vi "Commit Hardware Relay State.vi"(0 "RelayInterface in":refnum<class "RelayInterface.lvclass">, 5 "Session Handle in":T1, 11 "error in (no error)":errorcluster) -> (4 "RelayInterface out":refnum<class "RelayInterface.lvclass">, 15 "error out":errorcluster)   [LabVIEW 2015, in "RelayInterface.lvclass"]
uses:
  RelayInterface.lvclass
  SLSC Session/Typedefs/Session Handle.ctl
  SLSC Session/SLSC Session.lvclass
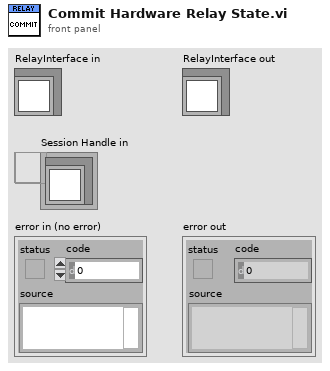
[diagram p1: front panel]
types:
  T1 = typedef "SLSC Switch.lvlib/SLSC Session.lvclass/Session Handle.ctl" = refnum<data-value>
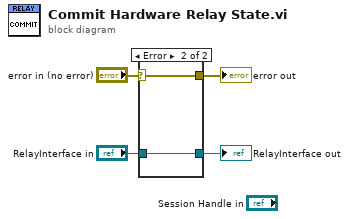
[diagram p0: block diagram]
diagram:
  n1 = case shown="Error" "error in (no error)" {
    selector: "error in (no error)" -> [w6 w8]
    tunnel: [w6 w8] -> w3
    tunnel: [w5 w7] -> w1
    tunnel: "RelayInterface in" -> [w5 w7]
    frame No Error {
    }
    frame Error {
    }
  }
  "error out" <- w3
  "RelayInterface out" <- w1
